vi "CRYGet Selected Channel Info.vi"(8 "In/out?":bool, 10 "Channel Name":string, 11 "Flattened Hardware":string) -> (0 "exist?":bool, 3 "Channel infor":T1={"ID"=0, "Name"="", "Digital"=FALSE, "Input"=FALSE, "Device Name"="", "Hardware Ch ID"=0, "Vmax (V)"=0.0, "Latency (samples)"=0.0, "Sampling Rate (Hz)"=0, "Bit Depth"=0, "Anti-aliasing Factor (%fs)"=0.475, "DAQmx Channel"="", "term config"=-1, "Coupling"=-1, "IEPE en"=FALSE, "ASIOChannel Name"="", "Audio Driver"=0, "ASIOChannel Index"=0} {"Coupling" items=["Default"=-1, "RSE"=10083, "NRSE"=10078, "Differential"=10106, "Pseudodifferential"=12529]; "term config" items=["Default"=-1, "RSE"=10083, "NRSE"=10078, "Differential"=10106, "Pseudodifferential"=12529]; "Anti-aliasing Factor (%fs)" format="%.2f"})   [LabVIEW 2013]
uses:
  Typedef Control/CRYHardware Channel Info.ctl
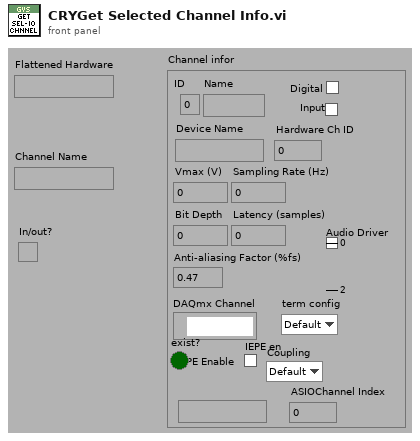
[diagram p1: front panel]
types:
  T1 = typedef "CRYHardware Channel Info.ctl" = cluster{"ID":i32, "Name":string, "Digital":bool, "Input":bool, "Device Name":string, "Hardware Ch ID":u8, "Vmax (V)":dbl, "Latency (samples)":dbl, "Sampling Rate (Hz)":u32, "Bit Depth":u32, "Anti-aliasing Factor (%fs)":sgl, "DAQmx Channel":tag, "term config":i32, "Coupling":i32, "IEPE en":bool, "ASIOChannel Name":string, "Audio Driver":u16, "ASIOChannel Index":u8}
  T2 = typedef "CRYHardware.ctl" = cluster{"Name":string, "Analog I/O":u16, "Digital I/O":u16, "Channels":u8, "Dig Dev ID":u8, "N ports":u8, "Interface":u32, "Dig I/O Ports":cluster{"port #":i16, "width":i16, "direction":i32}[], "Interf settings":cluster{"Type":u16, "COM Port":u8, "Baud rate":u32, "Data bits":u32, "Parity":u16, "Stop bits":u16, "Flow control":u16, "Dev ID IEEE":u8}[], "N interfs":i32, "udev SNs":i16[], "udev enable":bool, "Channel Array":T1[], "Cal sequence":string, "SelectedIn":u16, "SelectedOut":u16, "SelectedTab":u16, "State":bool, "Help":string, "Advanced":bool, "In Audio Driver":u16, "Out Audio Driver":u16}
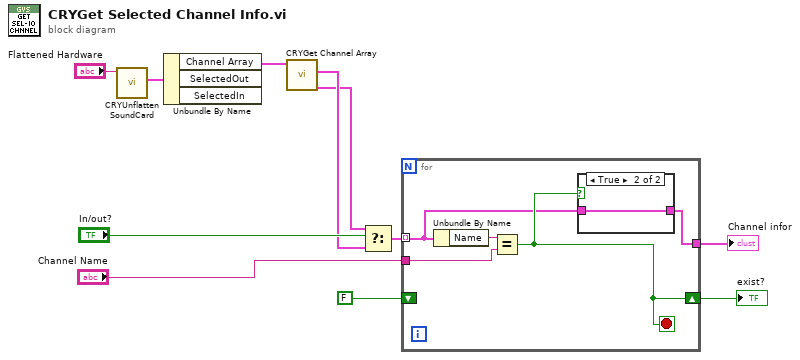
[diagram p0: block diagram]
diagram:
  n1 = call "CRYUnflatten SoundCard.vi"("Flatten SoundCard"="Flattened Hardware") -> ("SoundCard"=w11:T2)  [unwired: 10 out]
  n2 = Unbundle By Name(w11) -> ("Channel Array"=w10:T1[])  [unwired: 2 out]
  n3 = call "CRYGet Channel Array.vi"("Channel Array"=w10) -> ("I Channel Info Out"=w6:T1[], "O Channel Info Out"=w7:T1[])  [unwired: 9 out]
  n4 = Select(t=w6, s="In/out?", f=w7) -> (s? t:f=w5:T1[])
  n5 = for {
    tunnel: w5 -> [w13] mode=indexing
    tunnel: "Channel Name" -> [w15]
    shift-right: [w14] -> w2
    shift-left: FALSE ("x = y?") -> [_]
    tunnel: [w12] -> w1
    stop <- w14 stop-if-true
    n6 = Unbundle By Name(w13) -> ("Name"=w16:string)
    n7 = Equal?(x=w16, y=w15) -> (x = y?=w14:bool)
    n8 = case shown="True" w14 {
      tunnel: w13 -> [_ w17]
      tunnel: [_ w17] -> w12
      frame False {
      }
      frame True {
      }
    }
  }
  "Channel infor" <- w1
  "exist?" <- w2
